vi "Proceed.vi"(7 "component is ready (Y)":bool=TRUE, 8 "error in (no error)":errorcluster, 10 "ProceedMessage":refnum<class "ProceedMessage.lvclass">, 11 "RSA in":refnum<class "RSA.lvclass">) -> (0 "error out":errorcluster, 2 "all observers are ready?":bool, 3 "RSA out":refnum<class "RSA.lvclass">)   [LabVIEW 2012, in "RSA.lvclass"]
uses:
  RSA.lvclass
  <vilib>/Distrio/Murmex/ProceedMessage/ProceedMessage.lvclass
  <vilib>/Distrio/Murmex/GenericMessage/GenericMessage.lvclass
  RSA.lvclass/RSA.ctl
  <vilib>/Distrio/Murmex/ResetMessage/ResetMessage.lvclass
  <vilib>/Distrio/Murmex/StopMessage/StopMessage.lvclass
  <vilib>/Distrio/Murmex/Murmex/Murmex.lvclass
  <vilib>/Distrio/Murmex/Message/Add or replace parameter.vi
panel:
  # "This method is called when the PROCEED\ntrigger is sent. \n\nOverride this method when your component needs to\nrespond to this trigger. \n\nCall parent for proper implementation"
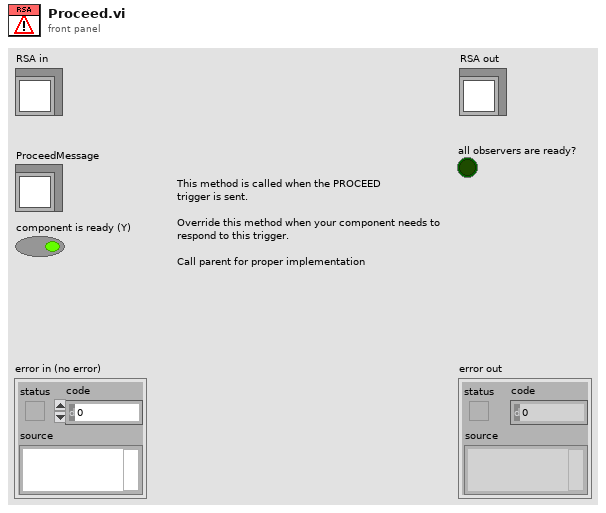
[diagram p1: front panel]
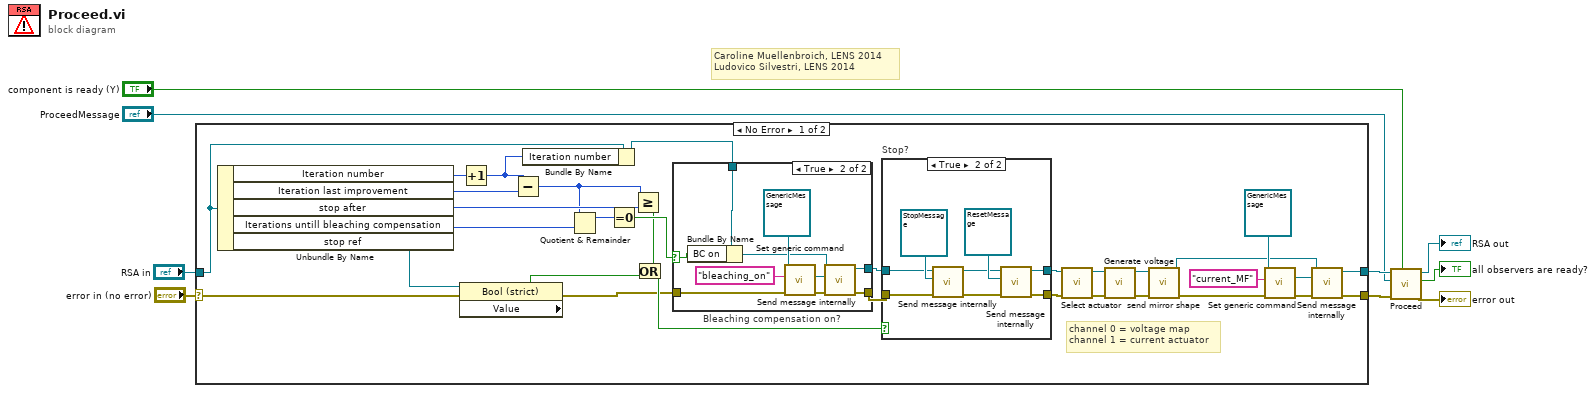
[diagram p0: block diagram]
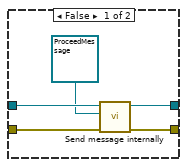
[diagram p3: hidden frame]
diagram:
  # "Caroline Muellenbroich, LENS 2014\nLudovico Silvestri, LENS 2014"
  n1 = case shown="No Error" "error in (no error)" {
    selector: "error in (no error)" -> [w10 w68]
    tunnel: [w17 w68] -> w5
    tunnel: "RSA in" -> [w27 w67]
    tunnel: [w16 w67] -> w2
    frame No Error {
      # "channel 0 = voltage map\nchannel 1 = current actuator"
      n2 = Unbundle By Name(w27) -> ("Iteration number"=w29:i32, "Iteration last improvement"=w38:i32, "stop after"=w41:i32, "Iterations untill bleaching compensation"=w35:i32, "stop ref"=w13:refnum<vi>)
      n3 = property class="Bool (strict)"(reference=w13, error in=w10) -> (error out=w11:errorcluster, "Value"=w12:bool)  [unwired: 1 out]
      n4 = Increment(x=w29) -> (x+1=w28:i32)
      n5 = Subtract(x=w28, y=w38) -> (x-y=w36:i32)
      n6 = Bundle By Name(cluster=w27, "Iteration number"=w28) -> (w26:refnum<class "RSA.lvclass">)
      n7 = Quotient & Remainder(x=w36, y=w35) -> (x-y*floor(x/y)=w34:i32)  [unwired: 1 out]
      n8 = Equal To 0?(x=w34) -> (x = 0?=w31:bool)
      n9 = Greater Or Equal?(x=w36, y=w41) -> (x >= y?=w15:bool)
      n10 = Or(x=w15, y=w12) -> (x .or. y?=w14:bool)
      n11 = case "Bleaching compensation on?" shown="True" w31 {
        selector: w31 -> [_ w44]
        tunnel: w26 -> [w43 w47]
        tunnel: [w43 w49] -> w39
        tunnel: w11 -> [w42 w50]
        tunnel: [w42 w48] -> w40
        frame False {
        }
        frame True {
          n12 = Bundle By Name(cluster=w47, "BC on"=w44) -> (w46:refnum<class "RSA.lvclass">)
          n13 = call <vilib>:"Set generic command.vi"("error in (no error)"=w50, "generic command"="bleaching_on", "GenericMessage in"=refnum<class "GenericMessage.lvclass"> refnum ("Murmex.lvlib:GenericMessage")) -> ("error out"=w52:errorcluster, "GenericMessage out"=w45:refnum<class "GenericMessage.lvclass">)  [unwired: 7 in]
          n14 = call <vilib>:"Send message internally.vi"("error in (no error)"=w52, "Message"=w45, "Murmex in"=w46) -> ("error out"=w48:errorcluster, "Murmex out"=w49:refnum<class "RSA.lvclass">)  [unwired: 7 in]
        }
      }
      n15 = case "Stop?" shown="True" w14 {
        tunnel: w40 -> [w58 w63]
        tunnel: w39 -> [w57 w60]
        tunnel: [w55 w66] -> w30
        tunnel: [w56 w65] -> w37
        frame False {
          n16 = call <vilib>:"Send message internally.vi"("error in (no error)"=w58, "Message"=refnum<class "ProceedMessage.lvclass"> refnum ("ProceedMessage"), "Murmex in"=w57) -> ("error out"=w56:errorcluster, "Murmex out"=w55:refnum<class "RSA.lvclass">)  [unwired: 7 in]
        }
        frame True {
          n17 = call <vilib>:"Send message internally.vi"("error in (no error)"=w63, "Message"=refnum<class "StopMessage.lvclass"> refnum ("Murmex.lvlib:StopMessage"), "Murmex in"=w60) -> ("error out"=w62:errorcluster, "Murmex out"=w59:refnum<class "RSA.lvclass">)  [unwired: 7 in]
          n18 = call <vilib>:"Send message internally.vi"("error in (no error)"=w62, "Message"=refnum<class "ResetMessage.lvclass"> refnum ("Message in"), "Murmex in"=w59) -> ("error out"=w65:errorcluster, "Murmex out"=w66:refnum<class "RSA.lvclass">)  [unwired: 7 in]
        }
      }
      n19 = call-dynamic "Select actuator.vi"("error in (no error)"=w37, "RSA in"=w30) -> ("error out"=w32:errorcluster, "RSA out"=w33:refnum<class "RSA.lvclass">)  [unwired: 8 in]
      n20 = call "Generate voltage.vi"("error in (no error)"=w32, "RSA in"=w33) -> ("error out"=w25:errorcluster, "RSA out"=w24:refnum<class "RSA.lvclass">)  [unwired: 8 in]
      n21 = call-dynamic "send mirror shape.vi"("error in (no error)"=w25, "RSA in"=w24) -> ("error out"=w21:errorcluster, "RSA out"=w19:refnum<class "RSA.lvclass">)  [unwired: 8 in]
      n22 = call <vilib>:"Set generic command.vi"("error in (no error)"=w21, "generic command"="current_MF", "GenericMessage in"=refnum<class "GenericMessage.lvclass"> refnum ("Murmex.lvlib:GenericMessage")) -> ("error out"=w22:errorcluster, "GenericMessage out"=w18:refnum<class "GenericMessage.lvclass">)  [unwired: 7 in]
      n23 = call <vilib>:"Send message internally.vi"("error in (no error)"=w22, "Message"=w18, "Murmex in"=w19) -> ("error out"=w17:errorcluster, "Murmex out"=w16:refnum<class "RSA.lvclass">)  [unwired: 7 in]
    }
    frame Error {
    }
  }
  n24 = call-parent "Proceed.vi"("component is ready (Y)"="component is ready (Y)", "error in (no error)"=w5, "ProceedMessage"="ProceedMessage", "Murmex in"=w2) -> ("error out"=→"error out":errorcluster, "all observers are ready?"=→"all observers are ready?":bool, "Murmex out"=→"RSA out":refnum<class "RSA.lvclass">)  [unwired: 5 in]
